vi "setcapacitor.vi"(1 "Characters to Write":string, 2 "GPIB\nAddress":string="1") -> (0 "Characters Read":string)   [LabVIEW 2019]
doc: "A device connected to a GPIB bus can be written to or be read from using this VI. Select the GPIB address of the device, choose Read or Write or both, type in the characters to be written, and run the VI. If you choose both Read and Write, the VI will write to the device first, then read from the device. Before using this VI you should initialize the GPIB address according to the device's specifications with the \"GPIB Initialization\" function."
panel:
  out "Write Status":string
  out "Read Status":string
  in  "# bytes\nto read":i32=200
  in  "Read":bool
  in  "Write":bool=TRUE
  # "Select  the GPIB address of the device, choose Read or Write or both, type in the characters to be written, and run the VI. If you choose both Read and Write, the VI will write to the device first, then read from the device.  Before using this VI, you should consider initializing the bus with the \"GPIB Initialization\" function."
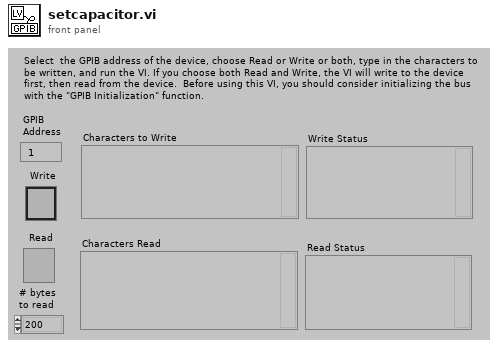
[diagram p1: front panel]
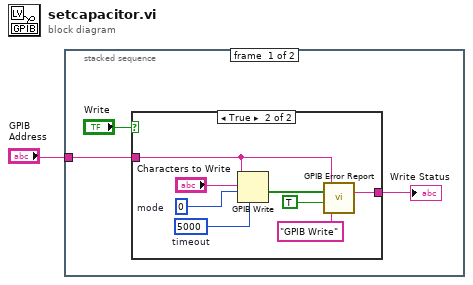
[diagram p0: block diagram]
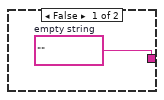
[diagram p2: hidden frame]
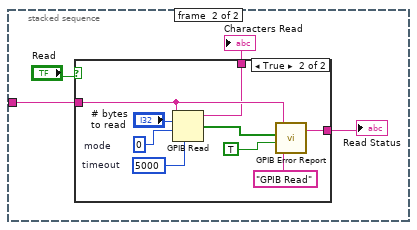
[diagram p3: hidden frame]
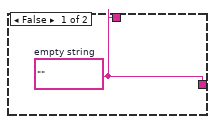
[diagram p4: hidden frame]
diagram:
  n1 = stacked-sequence {
    tunnel: "GPIB\nAddress" -> [w4 w17]
    frame #0 {
      n2 = case shown="True" "Write" {
        tunnel: [w5 w7] -> w2
        tunnel: w4 -> [_ w11]
        frame False {
          w5 = ""  # empty string
        }
        frame True {
          w13 = 0  # mode
          w6 = u32 5000  # timeout
          n3 = GPIB Write(0:w11, 1:"Characters to Write", 2:w13, 4:w6) -> (5:w10:bool[])  [unwired: 1 in, 1 out]
          n4 = call "GPIB Error Report.vi"("Function"="GPIB Write", "Dialog?(F)"=TRUE, "Status"=w10, "Address String"=w11) -> ("Status String"=w7:string)  [unwired: 1 out]
        }
      }
      "Write Status" <- w2
    }
    frame #1 {
      n5 = case shown="True" "Read" {
        tunnel: [w18 w21] -> w14
        tunnel: [w18 w22] -> w15
        tunnel: w17 -> [_ w26]
        frame False {
          w18 = ""  # empty string
        }
        frame True {
          w20 = u32 5000  # timeout
          w27 = 0  # mode
          n6 = GPIB Read(0:w26, 1:"# bytes\nto read", 2:w27, 4:w20) -> (5:w21:string, 6:w19:bool[])  [unwired: 1 in, 1 out]
          n7 = call "GPIB Error Report.vi"("Function"="GPIB Read", "Dialog?(F)"=TRUE, "Status"=w19, "Address String"=w26) -> ("Status String"=w22:string)  [unwired: 1 out]
        }
      }
      "Characters Read" <- w14
      "Read Status" <- w15
    }
  }
